vi "Pressure_Tubing_Correction.vi"(8 "Analogue In":dbl[][](array[numeric])) -> (0 "Analogue Out":dbl[][](array[numeric]))   [LabVIEW 2010]
uses:
  Globals/Constants_global.vi
  Globals/Meas_global.vi
  <vilib>/Analysis/2dsp.llb/Real FFT.vi
  <vilib>/Analysis/2dsp.llb/Inverse Real FFT.vi
  Globals/Dynamic_call_global.ph.vi
  <vilib>/Analysis/NI_AALPro.lvlib
panel:
  in  "Run?":bool=TRUE
  in  "Max.  Freq. required from ITF":dbl=10000.0
  out "Scanivalve_info":string
  out "Tubing Length":string
  out "Transfer Function":string
  out "Transducer\nZero Reading":dbl format="%#_p"
  out "Distorted Pressure Array Indicies":i32[](array[numeric])
  in  "Scani Valve?":bool
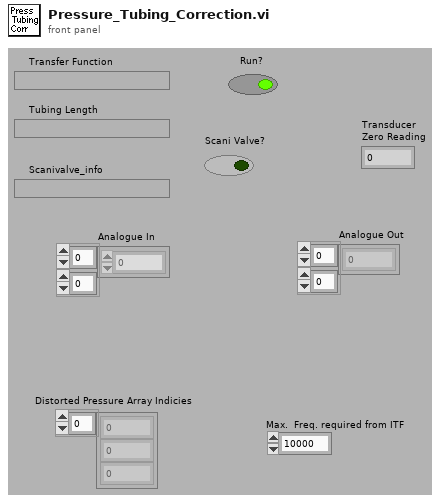
[diagram p1: front panel]
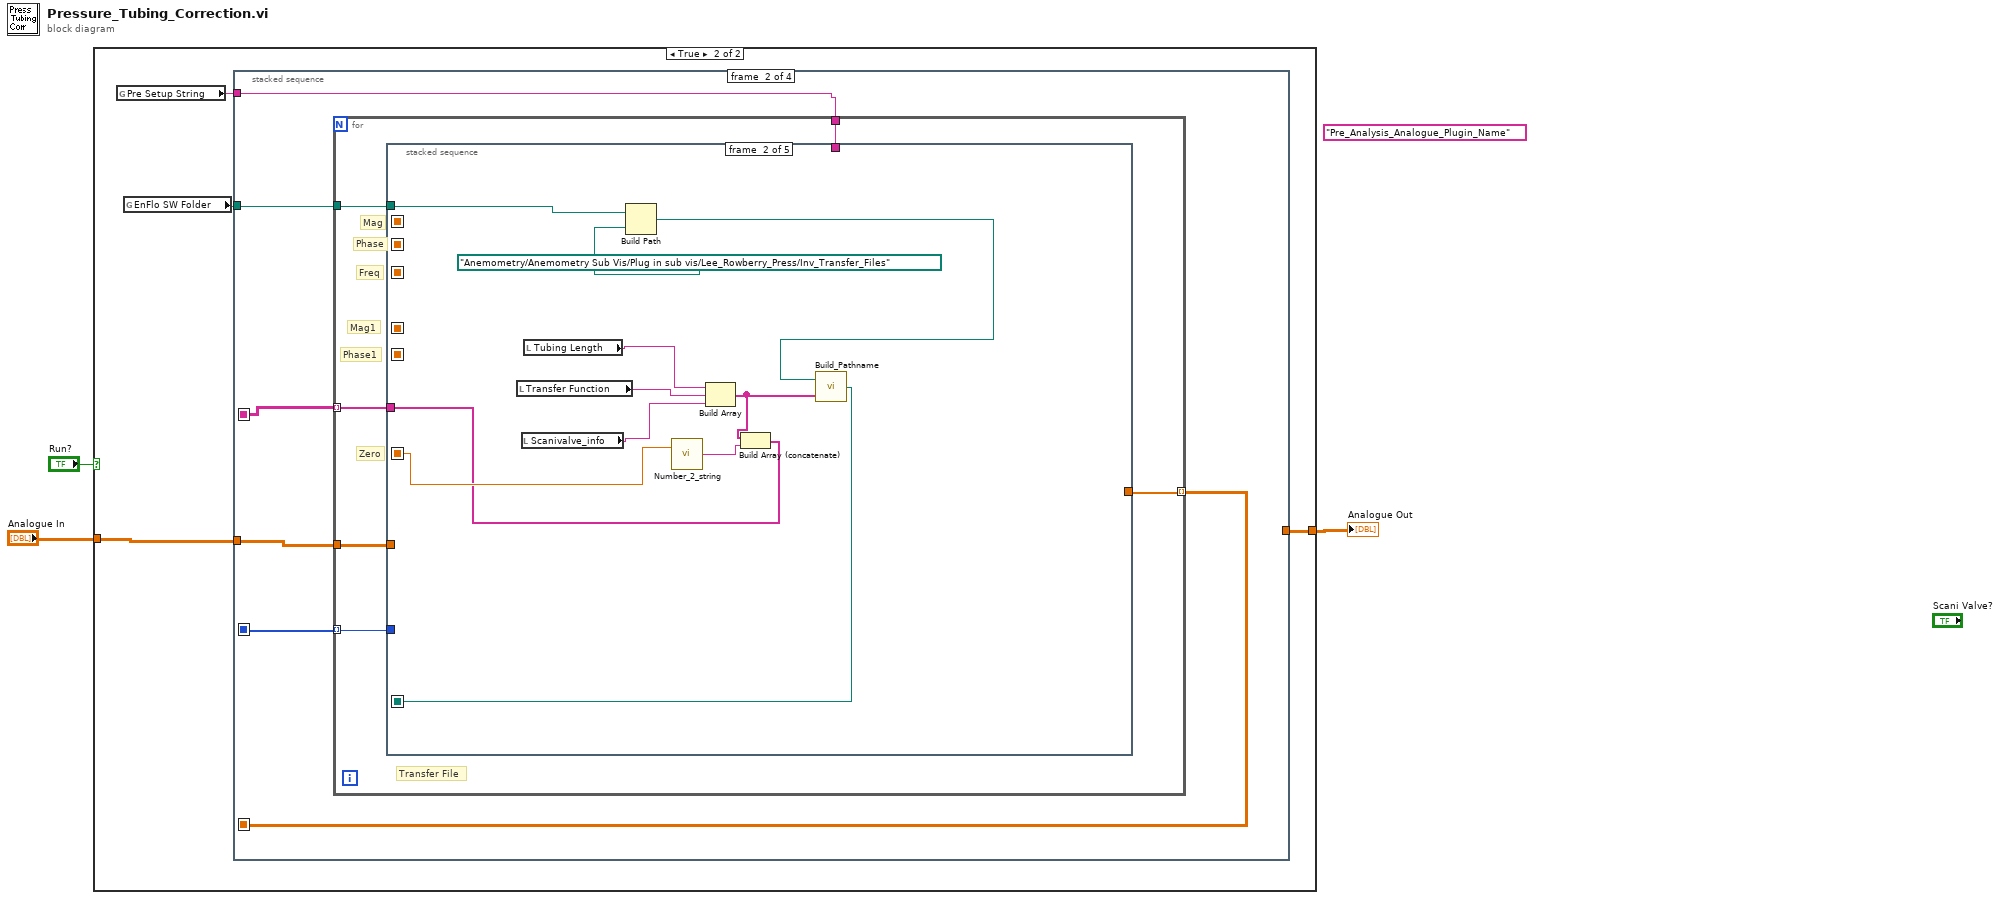
[diagram p0: block diagram]
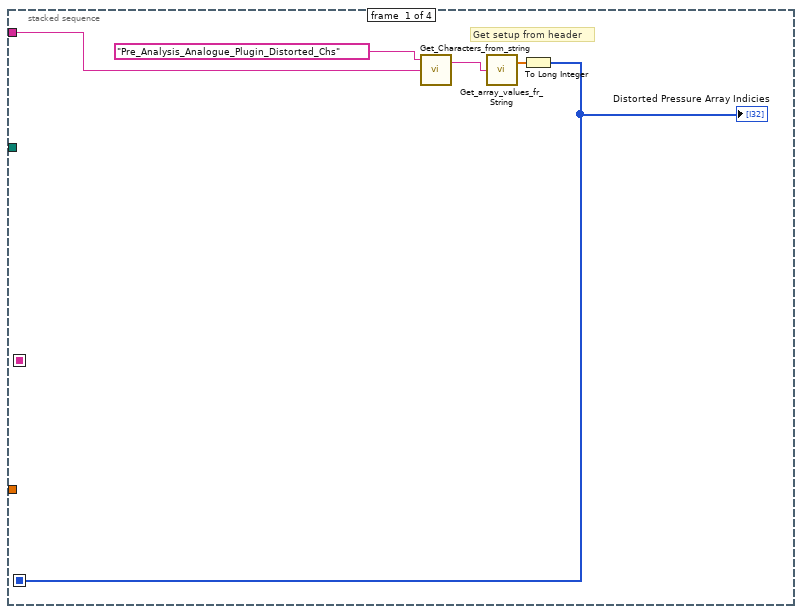
[diagram p3: hidden frame]
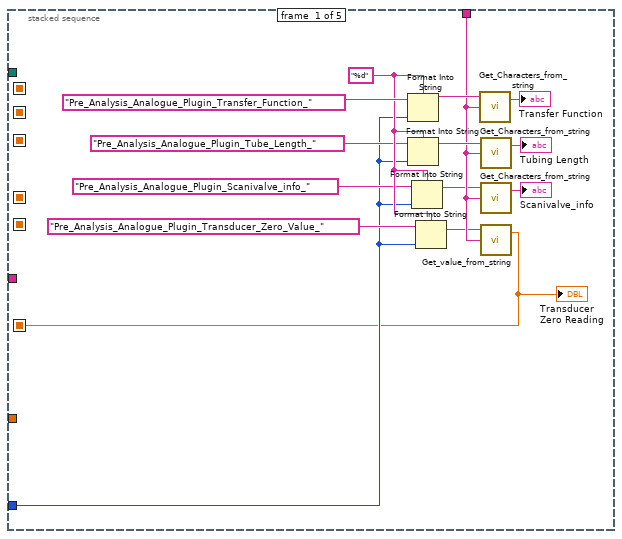
[diagram p4: hidden frame]
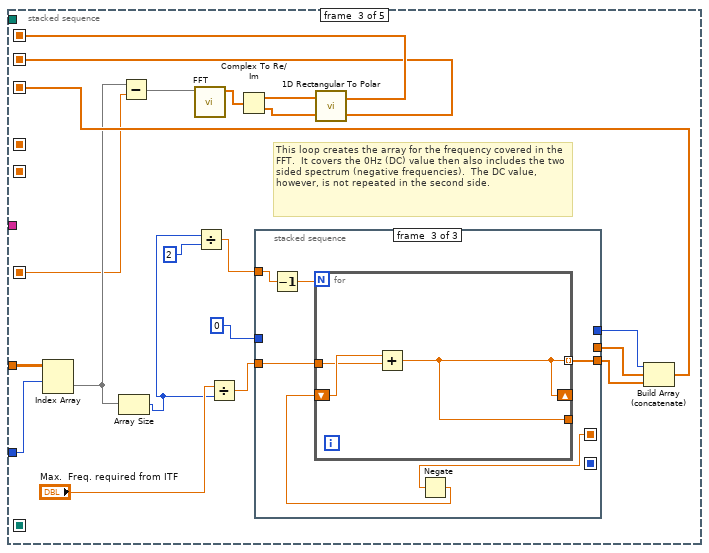
[diagram p5: hidden frame]
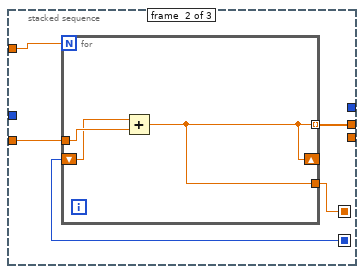
[diagram p7: hidden frame]
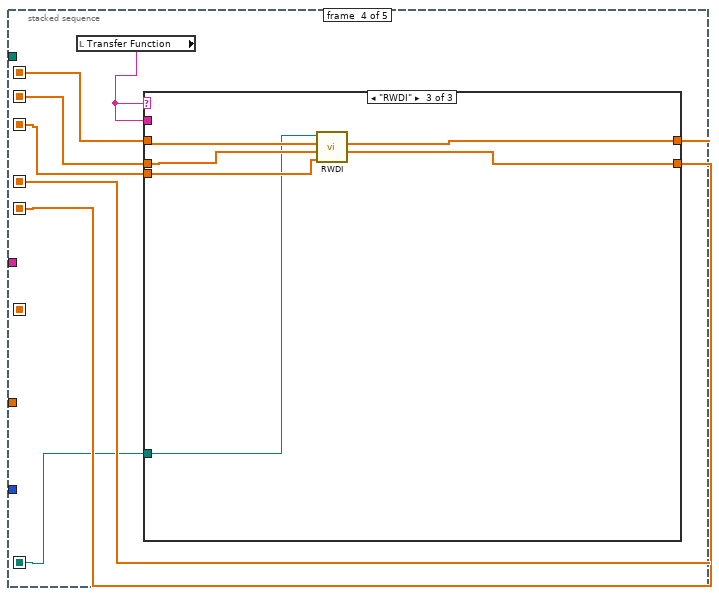
[diagram p8: hidden frame]
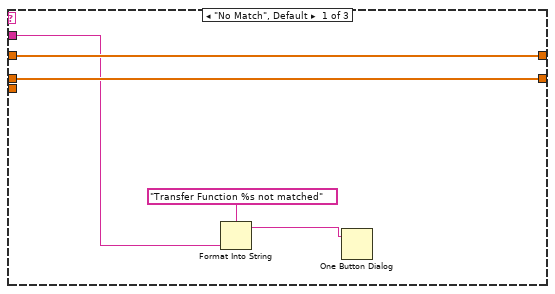
[diagram p9: hidden frame]
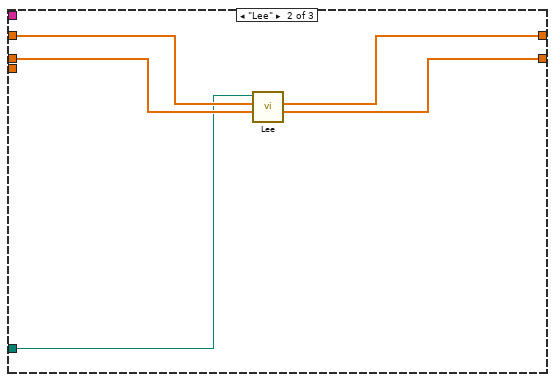
[diagram p10: hidden frame]
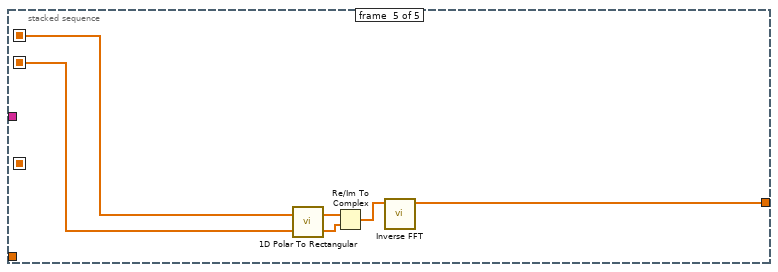
[diagram p11: hidden frame]
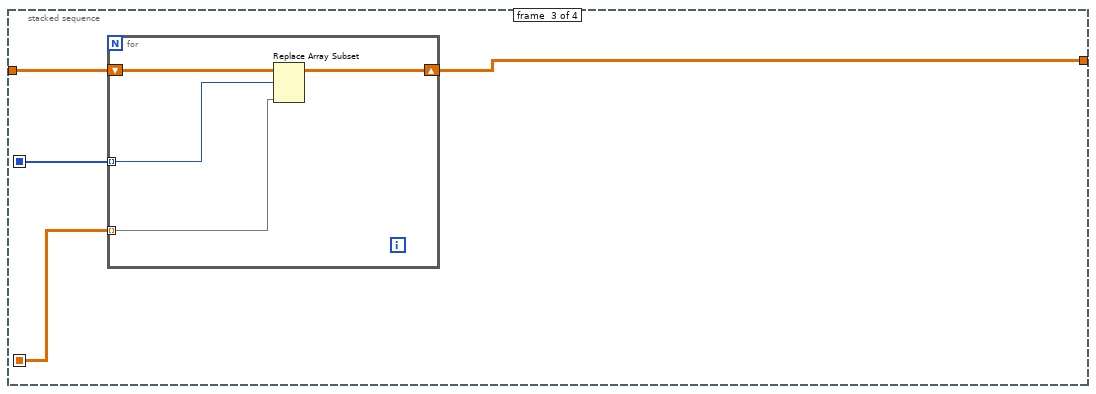
[diagram p12: hidden frame]
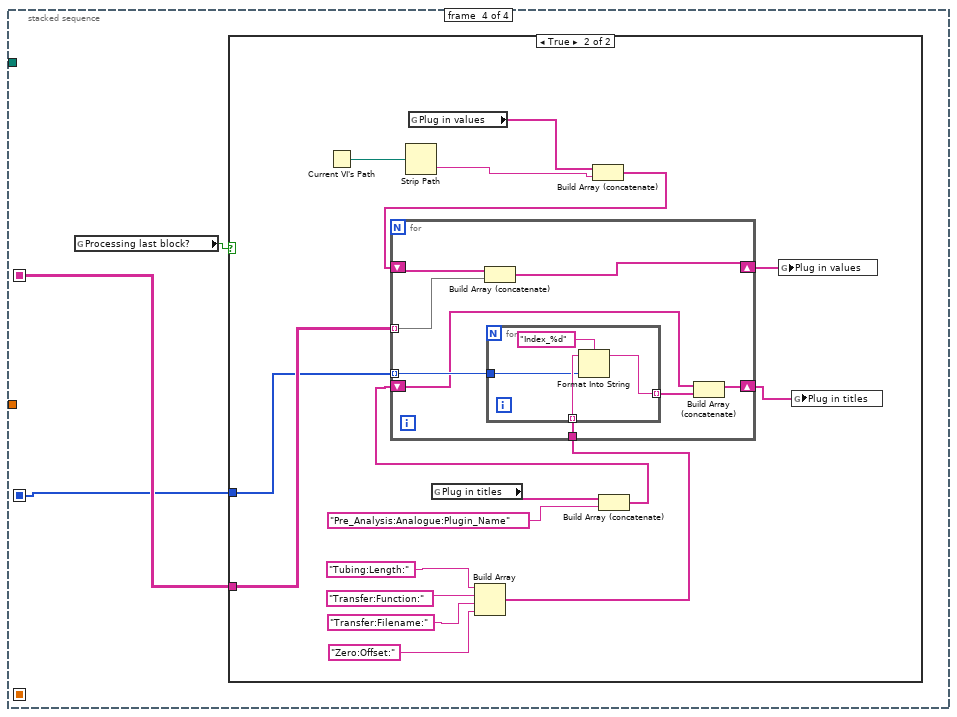
[diagram p13: hidden frame]
diagram:
  (unwired) "Pre_Analysis_Analogue_Plugin_Name"
  n1 = case shown="True" "Run?" {
    tunnel: "Analogue In" -> [w4 w7]
    tunnel: [w4 w5] -> w2
    frame False {
    }
    frame True {
      n2 = global read "Meas_global.vi" "Pre Setup String"() -> (w8:string)
      n3 = global read "Constants_global.vi" "EnFlo SW Folder"() -> (w6:path)
      n4 = stacked-sequence {
        seq-local: [w9 _ _ _] -> [_ w19 w121 w127]
        seq-local: [_ w16 _ _] -> [_ _ w120 _]
        seq-local: [_ w14 _ _] -> [_ _ _ w128]
        tunnel: w8 -> [w13 w18 _ _]
        tunnel: w6 -> [_ w17 _ _]
        tunnel: w7 -> [_ w15 w122 _]
        tunnel: [_ _ w119 _] -> w5
        frame #0 {
          # "Get setup from header"
          n5 = call "Get_Characters_from_string.vi"("Input string"=w13, "Variable name"="Pre_Analysis_Analogue_Plugin_Distorted_Chs") -> ("Value"=w11:string)  [unwired: 1 in, 1 out]
          n6 = call "Get_array_values_fr_String.vi"("String Value"=w11) -> ("Numeric Array"=w10:dbl[])  [unwired: 1 out]
          n7 = To Long Integer(number=w10) -> (32bit integer=w9:i32[])
          "Distorted Pressure Array Indicies" <- w9
        }
        frame #1 {
          n8 = for {
            tunnel: w15 -> [w25]
            tunnel: w19 -> [w24] mode=indexing
            tunnel: w18 -> [w23]
            tunnel: w17 -> [w22]
            tunnel: [w21] -> w16 mode=indexing
            tunnel: [w20] -> w14 mode=indexing
            # "Phase1"
            # "Mag1"
            # "Freq"
            # "Phase"
            # "Mag"
            # "Transfer File"
            # "Zero"
            n9 = stacked-sequence {
              seq-local: [w26 _ _ _ _] -> [_ w44 w53 _ _]
              seq-local: [_ w48 _ _ _] -> [_ _ _ w90 _]
              seq-local: [_ _ w63 _ _] -> [_ _ _ w95 _]
              seq-local: [_ _ w62 _ _] -> [_ _ _ w93 _]
              seq-local: [_ _ w61 _ _] -> [_ _ _ w91 _]
              seq-local: [_ _ _ w96 _] -> [_ _ _ _ w115]
              seq-local: [_ _ _ w94 _] -> [_ _ _ _ w114]
              tunnel: w25 -> [_ _ w59 _ _]
              tunnel: w24 -> [w27 _ w60 _ _]
              tunnel: w23 -> [w33 _ _ _ _]
              tunnel: w22 -> [_ w46 _ _ _]
              tunnel: [_ _ _ _ w113] -> w21
              tunnel: [_ w41 _ _ _] -> w20
              frame #0 {
                w38 = "%d" ("format string")
                n10 = Format Into String(format string=w38, initial string="Pre_Analysis_Analogue_Plugin_Transfer_Function_", w27) -> (resulting string=w39:string)  [unwired: 1 in, 1 out]
                n11 = Format Into String(format string=w38, initial string="Pre_Analysis_Analogue_Plugin_Tube_Length_", w27) -> (resulting string=w34:string)  [unwired: 1 in, 1 out]
                n12 = Format Into String(format string=w38, initial string="Pre_Analysis_Analogue_Plugin_Scanivalve_info_", w27) -> (resulting string=w31:string)  [unwired: 1 in, 1 out]
                n13 = Format Into String(format string=w38, initial string="Pre_Analysis_Analogue_Plugin_Transducer_Zero_Value_", w27) -> (resulting string=w32:string)  [unwired: 1 in, 1 out]
                n14 = call "Get_Characters_from_string.vi"("Input string"=w33, "Variable name"=w39) -> ("Value"=→"Transfer Function":string)  [unwired: 1 in, 1 out]
                n15 = call "Get_Characters_from_string.vi"("Input string"=w33, "Variable name"=w34) -> ("Value"=→"Tubing Length":string)  [unwired: 1 in, 1 out]
                n16 = call "Get_Characters_from_string.vi"("Input string"=w33, "Variable name"=w31) -> ("Value"=→"Scanivalve_info":string)  [unwired: 1 in, 1 out]
                n17 = call "Get_value_from_string.vi"("Input string"=w33, "Variable name"=w32) -> ("Value"=w26:dbl)  [unwired: 1 in, 1 out]
                "Transducer\nZero Reading" <- w26
              }
              frame #1 {
                n18 = local read "Transfer Function"() -> (w50:string)
                n19 = local read "Scanivalve_info"() -> (w49:string)
                n20 = local read "Tubing Length"() -> (w51:string)
                n21 = Build Path(base path=w46, name or relative path=path "Anemometry/Anemometry Sub Vis/Plug in sub vis/Lee_Rowberry_Press/Inv_Transfer_Files") -> (appended path=w45:path)
                n22 = call "Number_2_string.vi"("number"=w44) -> ("String"=w42:string)  [unwired: 1 in]
                n23 = Build Array(w51, w50, w49) -> (w43:string[])
                n24 = Build Array (concatenate)(w43, w42) -> (w41:string[])
                n25 = call "Build_Pathname.vi"("Output Array"=w43, "Pathname"=w45) -> ("Appended path"=w48:path)
              }
              frame #2 {
                # "This loop creates the array for the frequency covered in the FFT.  It covers the 0Hz (DC) value then also includes the two sided spectrum (negative frequencies).  The DC value, however, is not repeated in the second side."
                n26 = Index Array(array=w59, index (row)=w60) -> (element=w54:dbl[])  [unwired: 1 in]
                n27 = Array Size(array=w54) -> (size(s)=w55:i32)
                n28 = Subtract(x=w54, y=w53) -> (x-y=w52:dbl[])
                n29 = call-poly <vilib>:"FFT.vi"("X"=w52) -> ("FFT {X}"=w58:cdb[])  [unwired: 2 in, 8 out]
                n30 = Divide(x=w55, y=2) -> (x/y=w68:dbl)
                n31 = Divide(x="Max.  Freq. required from ITF", y=w55) -> (x/y=w66:dbl)
                n32 = Complex To Re/Im(x + iy=w58) -> (x=w57:dbl[], y=w56:dbl[])
                n33 = stacked-sequence {
                  seq-local: [w72 _ _] -> [_ w76 _]
                  seq-local: [_ w75 _] -> [_ _ w84]
                  tunnel: 0 -> [w72 _ _]
                  tunnel: w66 -> [_ w77 w86]
                  tunnel: w68 -> [_ w74 w82]
                  tunnel: [_ w73 _] -> w70
                  tunnel: [w72 _ _] -> w69
                  tunnel: [_ _ w85] -> w71
                  frame #0 {
                  }
                  frame #1 {
                    n34 = for {
                      N: w74 -> [_]
                      tunnel: w77 -> [w80]
                      tunnel: [w78] -> w73 mode=indexing
                      shift-right: [w78] -> _
                      shift-left: w76 -> [w79]
                      tunnel: [w78] -> w75
                      n35 = Add(x=w79, y=w80) -> (x+y=w78:dbl)
                    }
                  }
                  frame #2 {
                    n36 = Decrement(x=w82) -> (x-1=w81:dbl)
                    n37 = Negate(x=w84) -> (-x=w83:dbl)
                    n38 = for {
                      N: w81 -> [_]
                      tunnel: [w87] -> w85 mode=indexing
                      shift-right: [w87] -> _
                      shift-left: w83 -> [w89]
                      tunnel: [w87] -> _
                      tunnel: w86 -> [w88]
                      n39 = Add(x=w89, y=w88) -> (x+y=w87:dbl)
                    }
                  }
                }
                n40 = call <vilib>:"1D Rectangular To Polar.vi"("X"=w57, "Y"=w56) -> ("Magnitude"=w63:dbl[], "Phase"=w62:dbl[])  [unwired: 1 out]
                n41 = Build Array (concatenate)(w69, w70, w71) -> (w61:dbl[])
              }
              frame #3 {
                n42 = local read "Transfer Function"() -> (w92:string)
                n43 = case shown="\"RWDI\"" w92 {
                  tunnel: [w101 w104 w110] -> w96
                  tunnel: w95 -> [w101 w106 w112]
                  tunnel: [w100 w103 w109] -> w94
                  tunnel: w93 -> [w100 w105 w111]
                  tunnel: w92 -> [w99 _ _]
                  tunnel: w91 -> [_ _ w108]
                  tunnel: w90 -> [_ w102 w107]
                  frame "No Match", Default {
                    n44 = Format Into String(format string="Transfer Function %s not matched", w99) -> (resulting string=w97:string)  [unwired: 2 in, 1 out]
                    n45 = One Button Dialog(message=w97) -> ()  [unwired: 2 out]
                  }
                  frame "Lee" {
                    n46 = call "Lee.vi"("Phase In"=w105, "Magnitude In"=w106, "Tranfer_Function_File"=w102) -> ("Phase Out"=w103:dbl[], "Magnitude Out"=w104:dbl[])  [unwired: 1 in, 2 out]
                  }
                  frame "RWDI" {
                    n47 = call "RWDI.vi"("Freq"=w108, "Phase In"=w111, "Magnitude In"=w112, "Tranfer_Function_File"=w107) -> ("Phase Out"=w109:dbl[], "Magnitude Out"=w110:dbl[])  [unwired: 2 out]
                  }
                }
              }
              frame #4 {
                n48 = call <vilib>:"1D Polar To Rectangular.vi"("Magnitude"=w115, "Phase"=w114) -> ("X"=w118:dbl[], "Y"=w116:dbl[])  [unwired: 1 out]
                n49 = Re/Im To Complex(1:w116, 2:w118) -> (0:w117:cdb[])
                n50 = call-poly <vilib>:"Inverse FFT.vi"("FFT {X}"=w117) -> ("X"=w113:dbl[])  [unwired: 1 in, 9 out]
              }
            }
          }
        }
        frame #2 {
          n51 = for {
            shift-right: [w123] -> w119
            shift-left: w122 -> [w124]
            tunnel: w121 -> [w126] mode=indexing
            tunnel: w120 -> [w125] mode=indexing
            n52 = Replace Array Subset(array=w124, new element=w125, index (row)=w126) -> (w123:dbl[][])  [unwired: 1 in]
          }
        }
        frame #3 {
          n53 = global read "Meas_global.vi" "Processing last block?"() -> (w129:bool)
          n54 = case shown="True" w129 {
            tunnel: w128 -> [_ w139]
            tunnel: w127 -> [_ w132]
            frame False {
            }
            frame True {
              n55 = Current VI's Path() -> (path=w142:path)
              n56 = Strip Path(path=w142) -> (name=w141:string)  [unwired: 1 out]
              n57 = global read "Dynamic_call_global.ph.vi" "Plug in values"() -> (w145:string[])
              n58 = global read "Dynamic_call_global.ph.vi" "Plug in titles"() -> (w144:string[])
              n59 = Build Array("Tubing:Length:", "Transfer:Function:", "Transfer:Filename:", "Zero:Offset:") -> (w133:string[])
              n60 = Build Array (concatenate)(w145, w141) -> (w140:string[])
              n61 = Build Array (concatenate)(w144, "Pre_Analysis:Analogue:Plugin_Name") -> (w137:string[])
              n62 = for {
                shift-right: [w151] -> w138
                shift-left: w140 -> [w153]
                shift-right: [w146] -> w131
                shift-left: w137 -> [w148]
                tunnel: w139 -> [w152] mode=indexing
                tunnel: w133 -> [w150]
                tunnel: w132 -> [w149] mode=indexing
                n63 = Build Array (concatenate)(w153, w152) -> (w151:string[])
                n64 = for {
                  tunnel: w150 -> [w157] mode=indexing
                  tunnel: w149 -> [w156]
                  tunnel: [w154] -> w147 mode=indexing
                  n65 = Format Into String(format string="Index_%d", initial string=w157, w156) -> (resulting string=w154:string)  [unwired: 1 in, 1 out]
                }
                n66 = Build Array (concatenate)(w148, w147) -> (w146:string[])
              }
              n67 = global write "Dynamic_call_global.ph.vi" "Plug in values"(w138) -> ()
              n68 = global write "Dynamic_call_global.ph.vi" "Plug in titles"(w131) -> ()
            }
          }
        }
      }
    }
  }
  "Analogue Out" <- w2
